vi "CR-字符检测处理函数1.vi"(8 "error in (no error)":errorcluster caption="错误输入（无错误）", 10 "CR- 字符检测参数 2":T4={"File Path (字符库)"=path "D:/Inspect System/Source Code/Template Program/字符模板.abc", "Url"="http://10.6.1.31:8080/MesInnerpackLineIO.asmx", "accessKey"="a45b2d3334ffs_\na45b2d3334ffs_", "字符长度设定"=0, "File Path (连接件模板)"=path "D:/Inspect System/Source Code/Template Program/字符检测定位模板.png", "Parameters (OCR/OCV 1)"={"Threshold Data"={"Method"=enum."Local", "Looking for"=1, "Color Mode"=0, "Kernel Size"={"Width"=32, "Height"=32}, "Ranges"=[{"Min"=1, "Max"=255}]}, "Reject Border"=TRUE, "Number Of Erosions"=0, "Size & Spacing"={"Segment Algorithm"=0, "Min Bounding Rect Width"=1, "Max Bounding Rect Width"=65536, "Min Bounding Rect Height"=1, "Max Bounding Rect Height"=65536, "Min Character Size"=20, "Max Character Size"=65536, "Min Char Spacing"=1, "Max Horiz Element Spacing"=1, "Max Vert Element Spacing"=0, "Max Space Distance"=65536}, "Read Options"={"Read Strategy"=1, "Read Resolution"=2, "Scale Dependant"=FALSE, "Aspect Ratio"=400, "Acceptance Level"=700, "Substitution Character"="?", "MultiLine"=TRUE}, "Valid Characters"=[], "Use Text Pattern"=FALSE, "Orientation"=0, "# Lines Expected"=0, "Number of Blocks"=4}, "Rectangle"={"Left"=0, "Top"=0, "Right"=0, "Bottom"=0, "Rotation"=0.0}} {"Rectangle"."Rotation" min=-90.0 max=90.0 step=1.0 format="%.2f"; "Rectangle"."Left" scale=0.0..1024.0; "Rectangle"."Right" scale=0.0..1024.0; "Parameters (OCR/OCV 1)"."Threshold Data"."Looking for" items=["Light on Dark", "Dark on Light"]; "Parameters (OCR/OCV 1)"."Threshold Data"."Color Mode" items=["RGB", "HSL", "HSV", "HSI"]; "Parameters (OCR/OCV 1)"."Size & Spacing"."Segment Algorithm" items=["None", "Shortest Segment", "Legacy Auto Split"]; "Parameters (OCR/OCV 1)"."Read Options"."Read Strategy" items=["Aggressive", "Conservative"]; "Parameters (OCR/OCV 1)"."Read Options"."Read Resolution" items=["Low", "Medium", "High"]; "Parameters (OCR/OCV 1)"."Valid Characters"."Pre-defined characters" items=["Any Character", "User-defined Characters", "Alphabetic", "Alphanumeric", "Uppercase Letters", "Lowercase Letters", "Decimal Digits", "Hexadecimal Digits", "Pattern", "Force Space"]; "Parameters (OCR/OCV 1)"."Orientation" items=["Baseline inside", "Baseline outside"]}, 11 "Image in":T5(plugin-control)) -> (0 "error out":errorcluster caption="错误输出", 1 "布尔":bool, 2 "String (OCR/OCV 1)":string, 3 "Image out":T5(plugin-control), 5 "模板匹配OK/NG":bool)   [LabVIEW 2017]
uses:
  <vilib>/vision/NI_Vision_Development_Module.lvlib
panel:
  in  "Coordinate System Out":T1 {"Measurement System"."Axis Reference" items=["Direct", "Indirect"]; "Measurement System"."Angle (deg)" format="%.2f"; "Measurement System"."Origin"."Y" format="%.2f"; "Measurement System"."Origin"."X" format="%.2f"; "Reference System"."Axis Reference" items=["Direct", "Indirect"]; "Reference System"."Angle (deg)" format="%.2f"; "Reference System"."Origin"."Y" format="%.2f"; "Reference System"."Origin"."X" format="%.2f"}
  in  "Parameters (Pattern Matching 1)":T2={"Number of Matches Requested"=1, "Minimum Match Score"=500.0, "Angle Ranges"=[{"Start Angle"=-45.0, "End Angle"=45.0}, {"Start Angle"=135.0, "End Angle"=225.0}]}
  out "Number of Matches (Geometric Matching 1)":i32
  out "长度":i32
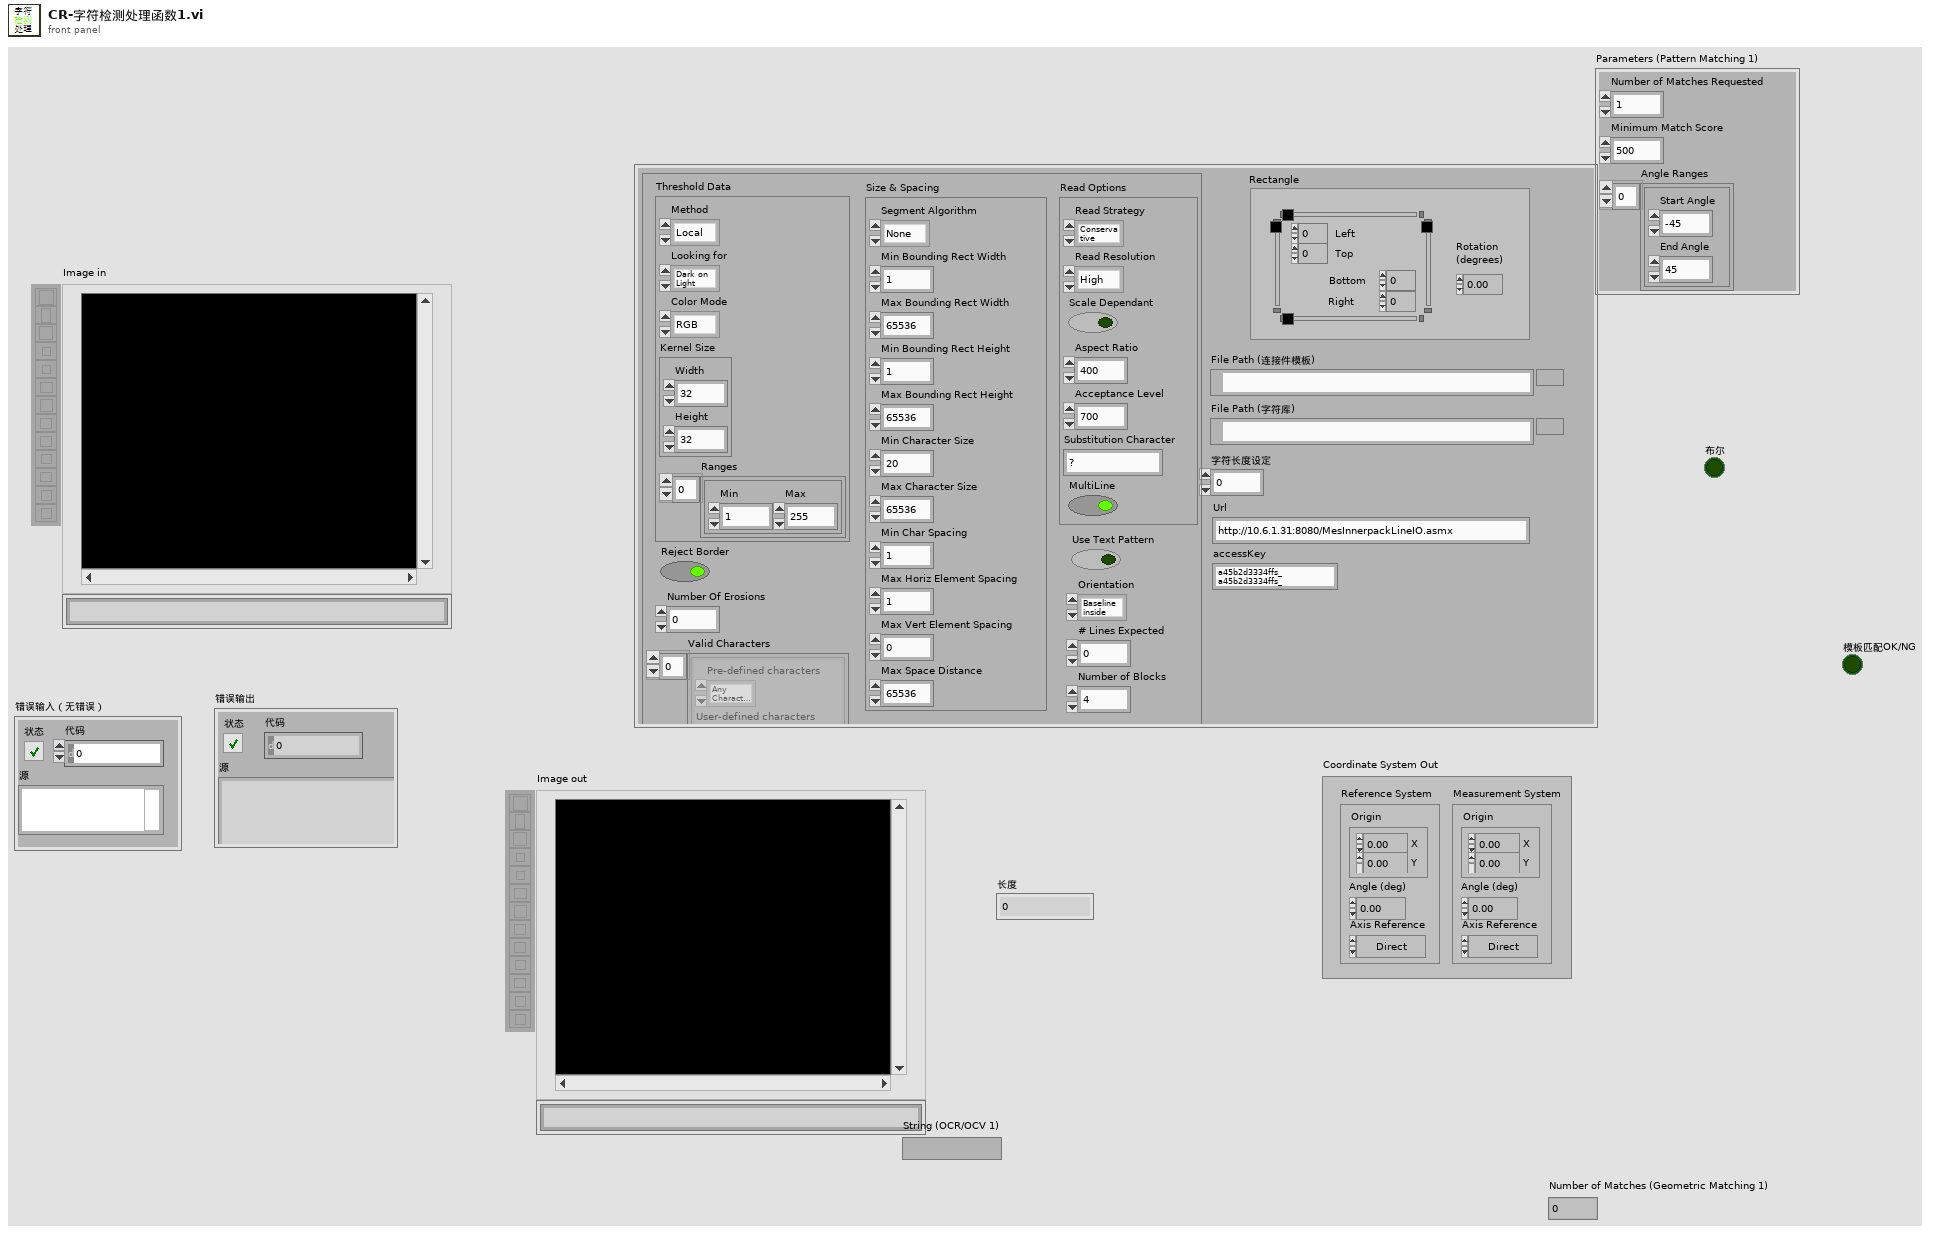
[diagram p1: front panel]
types:
  T1 = typedef "IMAQ Coordinate System" = cluster{"Reference System":cluster{"Origin":cluster{"X":sgl, "Y":sgl}, "Angle (deg)":sgl, "Axis Reference":u32}, "Measurement System":cluster{"Origin":cluster{"X":sgl, "Y":sgl}, "Angle (deg)":sgl, "Axis Reference":u32}}
  T2 = cluster{"Number of Matches Requested":i32, "Minimum Match Score":sgl, "Angle Ranges":cluster{"Start Angle":sgl, "End Angle":sgl}[]}
  T3 = typedef "IMAQ Rectangle" = cluster{"Left":i32, "Top":i32, "Right":i32, "Bottom":i32, "Rotation":dbl}
  T4 = cluster{"File Path (字符库)":path, "Url":string, "accessKey":string, "字符长度设定":i32, "File Path (连接件模板)":path, "Parameters (OCR/OCV 1)":cluster{"Threshold Data":cluster{"Method":enum16{"Fixed Range", "Uniform", "Linear", "Non Linear", "Local", "Color"}, "Looking for":u32, "Color Mode":u32, "Kernel Size":cluster{"Width":i32, "Height":i32}, "Ranges":cluster{"Min":i32, "Max":i32}[]}, "Reject Border":bool, "Number Of Erosions":i32, "Size & Spacing":cluster{"Segment Algorithm":u16, "Min Bounding Rect Width":i32, "Max Bounding Rect Width":i32, "Min Bounding Rect Height":i32, "Max Bounding Rect Height":i32, "Min Character Size":i32, "Max Character Size":i32, "Min Char Spacing":i32, "Max Horiz Element Spacing":i32, "Max Vert Element Spacing":i32, "Max Space Distance":i32}, "Read Options":cluster{"Read Strategy":i32, "Read Resolution":i32, "Scale Dependant":bool, "Aspect Ratio":i32, "Acceptance Level":i32, "Substitution Character":string, "MultiLine":bool}, "Valid Characters":cluster{"Pre-defined characters":i32, "User-defined characters":string}[], "Use Text Pattern":bool, "Orientation":u32, "# Lines Expected":u32, "Number of Blocks":i32}, "Rectangle":T3}
  T5 = typedef "IMAQ Image.ctl" = refnum<image>
  T6 = cluster{"Left":i32, "Top":i32, "Right":i32, "Bottom":i32}
  T7 = typedef "ROI Descriptor" = cluster{"Global Rectangle":i32[], "Contours":cluster{"ID":enum32{"External", "Internal"}, "Type":u32, "Coordinates":i32[]}[]}
  T8 = cluster{"Origin":cluster{"X":sgl, "Y":sgl}, "Angle (deg)":sgl, "Axis Reference":u32}
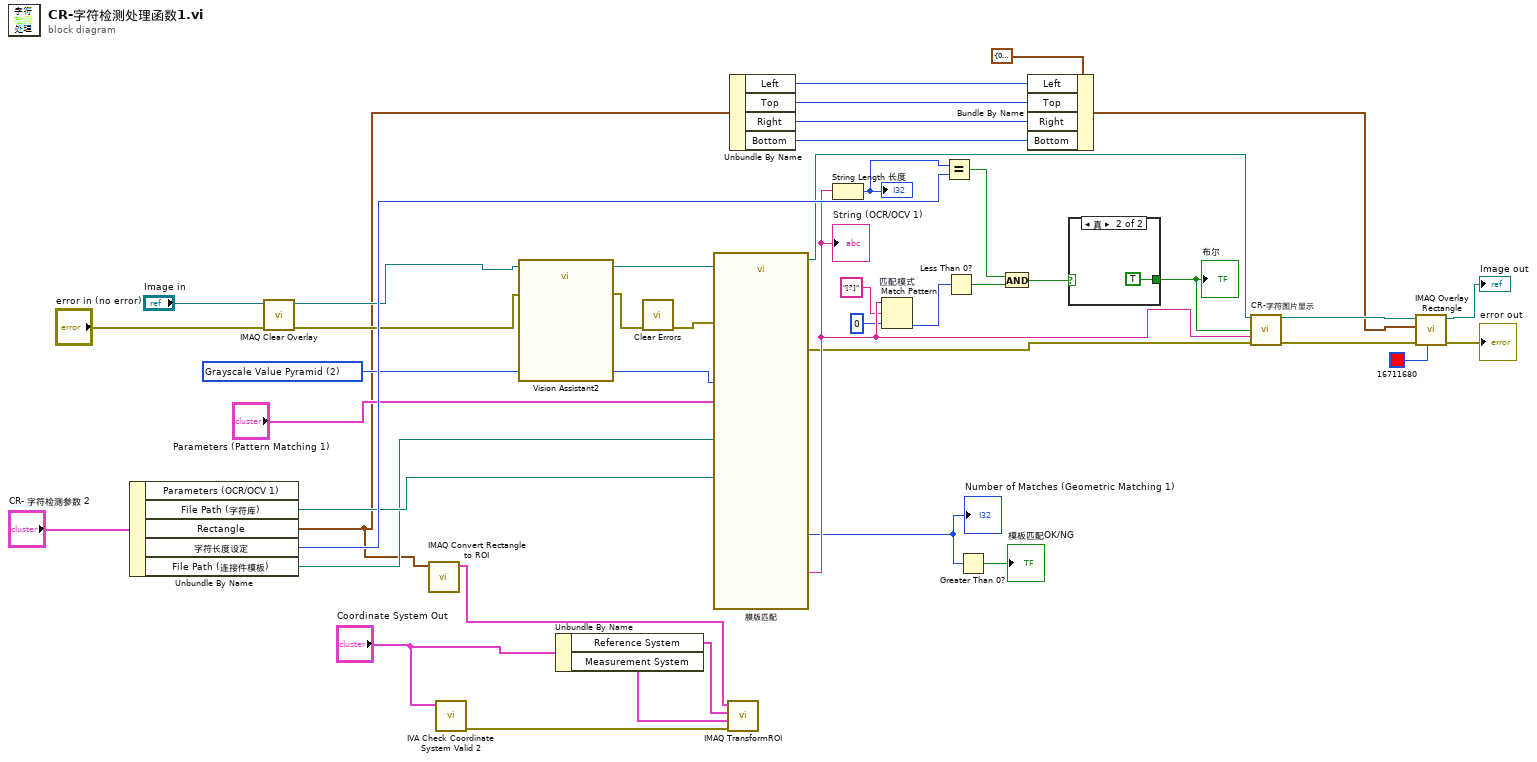
[diagram p0: block diagram]
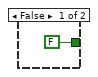
[diagram p2: hidden frame]
diagram:
  w16 = 2 items=["All", "Low Discrepancy Sampling", "Grayscale Value Pyramid", "Gradients Pyramid"] ("Algorithm (Pattern Matching 1)")
  n1 = Unbundle By Name("CR- 字符检测参数 2") -> ("File Path (字符库)"=w37:path, "Rectangle"=w6:T3, "字符长度设定"=w40:i32, "File Path (连接件模板)"=w24:path)  [unwired: 1 out]
  n2 = call "IMAQ Clear Overlay"("error in (no error)"="error in (no error)", "Image"="Image in") -> ("error out"=w10:errorcluster, "Image Out"=w12:T5)  [unwired: 8 in]
  n3 = call "IMAQ Convert Rectangle to ROI"("Rectangle"=w6) -> ("ROI Descriptor"=w5:T7)  [unwired: 8 in, 1 out]
  n4 = call <vilib>:"IVA Check Coordinate System Valid 2.vi"("Coordinate System"="Coordinate System Out") -> ("error out"=w4:errorcluster)  [unwired: 1 in, 9 out]
  n5 = call "Vision Assistant2"("Image In"=w12, "error in"=w10) -> ("Image Out"=w11:T5, "error out"=w9:errorcluster)  [unwired: 22 in, 2 out]
  n6 = Unbundle By Name("Coordinate System Out") -> ("Reference System"=w3:T8, "Measurement System"=w2:T8)
  n7 = call <vilib>:"Clear Errors.vi"("error in (no error)"=w9) -> ("error out"=w7:errorcluster)  [unwired: 5 in, 1 out]
  n8 = call "膜版匹配.vi"("Image In"=w11, "Algorithm (Pattern Matching 1)"=w16, "Parameters (Pattern Matching 1)"="Parameters (Pattern Matching 1)", "Template File Path (Pattern Matching 1)"=w24, "error in"=w7, "File Path (OCR/OCV 1)"=w37) -> ("Image Out"=w38:T5, "String (OCR/OCV 1)"=w36:string, "Number of Matches (Pattern Matching 1)"=w35:i32, "error out"=w8:errorcluster)  [unwired: 15 in, 3 out]
  "String (OCR/OCV 1)" <- w36
  "Number of Matches (Geometric Matching 1)" <- w35
  n9 = call "IMAQ TransformROI"("error in (no error)"=w4, "New Reference"=w2, "Base Reference"=w3, "ROI Descriptor"=w5) -> ()  [unwired: 8 out]
  n10 = Unbundle By Name(w6) -> ("Left"=w32:i32, "Top"=w31:i32, "Right"=w30:i32, "Bottom"=w29:i32)
  n11 = String Length(string=w36) -> (length=w22:i32)
  "长度" <- w22
  n12 = Match Pattern "匹配模式"(string=w36, regular expression="[?]" ("正则表达式"), offset (0)=0 ("偏移量(0)")) -> (offset past match=w19:i32)  [unwired: 3 out]
  n13 = Equal?(x=w22, y=w40) -> (x = y?=w17:bool)
  n14 = Less Than 0?(x=w19) -> (x < 0?=w18:bool)
  n15 = Greater Than 0?(x=w35) -> (x > 0?=→"模板匹配OK/NG":bool)
  n16 = And(x=w17, y=w18) -> (x .and. y?=w39:bool)
  n17 = Bundle By Name(cluster=T6 {"Left"=0, "Top"=0, "Right"=0, "Bottom"=0} ("Rectangle"), "Left"=w32, "Top"=w31, "Right"=w30, "Bottom"=w29) -> (w28:T6)
  n18 = case shown="真" w39 {
    tunnel: [FALSE TRUE] -> w41
    frame False {
    }
    frame True {
    }
  }
  "布尔" <- w41
  n19 = call "CR-字符图片显示.vi"("Image in"=w38, "是否检测到字符串"=w41, "String (OCR/OCV 1)"=w36, "error in (no error)"=w8) -> ("Image out"=w42:T5, "error out"=w27:errorcluster)  [unwired: 10 in]
  n20 = call "IMAQ Overlay Rectangle"("Color"=u32 16711680, "error in (no error)"=w27, "Rectangle"=w28, "Image"=w42) -> ("error out"=→"error out":errorcluster, "Image Out"=→"Image out":T5)  [unwired: 6 in]
